vi "Resume UI Updates.vi"(8 "error in":errorcluster, 11 "Module Data":T1) -> (0 "error out":errorcluster, 3 "Module Data":T1)   [LabVIEW 2020, in "Peek Window.lvlib"]
uses:
  Peek Window.lvlib
  MHL Data Cluster.ctl
  VI Types/Standard VI Type/Standard VI Type.lvclass
  Open Diagram Argument--cluster.ctl
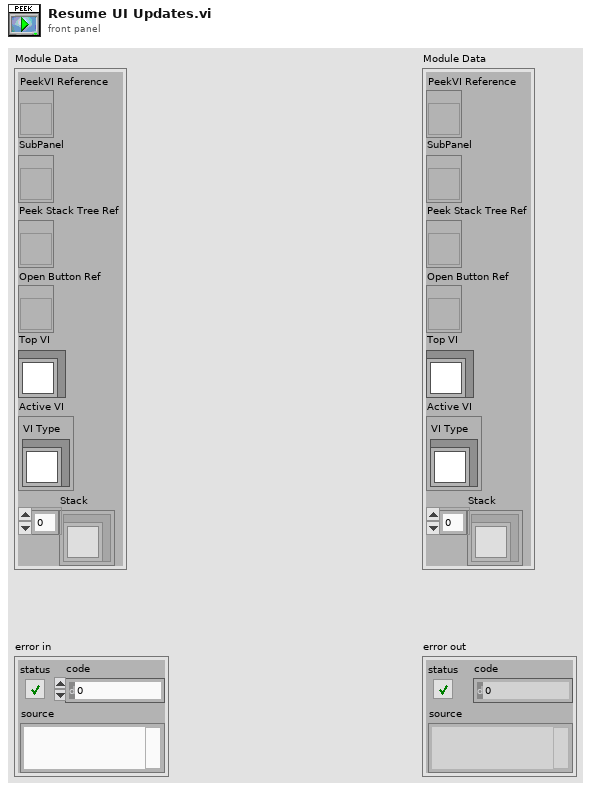
[diagram p1: front panel]
types:
  T1 = typedef "Peek Window.lvlib/MHL Data Cluster.ctl" = cluster{"PeekVI Reference":refnum<vi>, "SubPanel":refnum<vi>, "Peek Stack Tree Ref":refnum<vi>, "Open Button Ref":refnum<vi>, "Top VI":refnum<class "Standard VI Type.lvclass">, "Active VI":T2, "Stack":refnum<class "Standard VI Type.lvclass">[]}
  T2 = typedef "Peek Window.lvlib/Open Diagram Argument--cluster.ctl" = cluster{"VI Type":refnum<class "Standard VI Type.lvclass">}
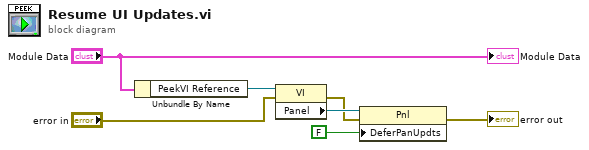
[diagram p0: block diagram]
diagram:
  n1 = Unbundle By Name("Module Data") -> ("PeekVI Reference"=w7:refnum<vi>)
  n2 = property class="VI"(reference=w7, error in="error in") -> (error out=w5:errorcluster, "Panel"=w6:refnum<vi>)  [unwired: 1 out]
  n3 = property class="Pnl"(reference=w6, error in=w5, "DeferPanUpdts"=FALSE) -> (error out=→"error out":errorcluster)  [unwired: 1 out]
  "Module Data" <- "Module Data"
